vi "StoreAction.vi"(7 "Enum":enum16{"Set", "Get"}(ring)=enum."Get", 8 "Error in":errorcluster, 11 "Write action":string) -> (0 "Error out":errorcluster, 3 "Read action":string)   [LabVIEW 2017]
doc: "This functional global is used to store the action which needs to be taken when the enter button is pressed"
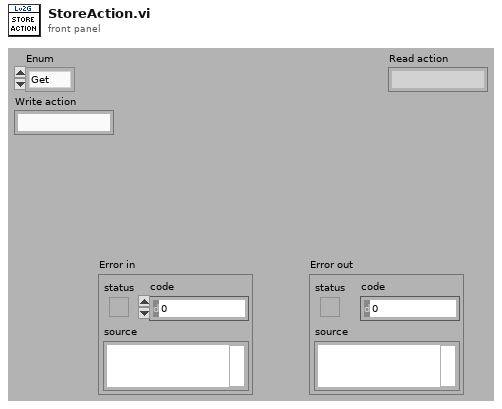
[diagram p1: front panel]
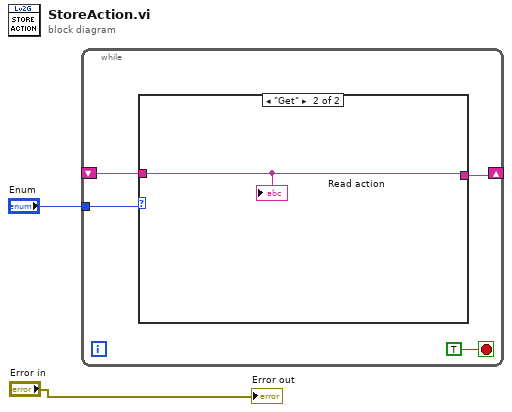
[diagram p0: block diagram]
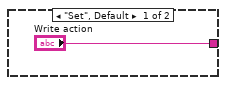
[diagram p2: hidden frame]
diagram:
  n1 = while {
    tunnel: "Enum" -> [w6]
    shift-right: [w5] -> _
    shift-left: _ -> [w4]
    stop <- TRUE stop-if-true
    n2 = case shown="\"Get\"" w6 {
      tunnel: ["Write action" w8] -> w5
      tunnel: w4 -> [_ w8]
      frame "Set", Default {
      }
      frame "Get" {
        "Read action" <- w8
      }
    }
  }
  "Error out" <- "Error in"
